vi "Feeder Move Arms.vi"(8 "error in (no error)":errorcluster, 11 "Action":enum16{"Drop", "Lift"}(ring)=enum."Lift") -> (0 "error out":errorcluster)   [LabVIEW 2014]
uses:
  Main/Robot Global Data.vi
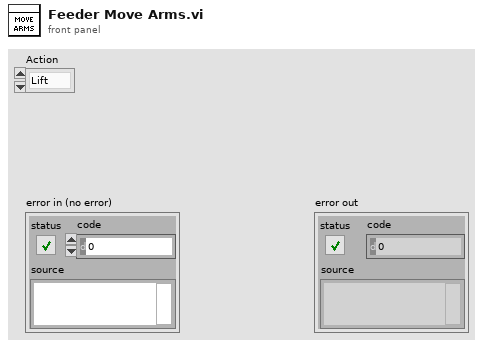
[diagram p1: front panel]
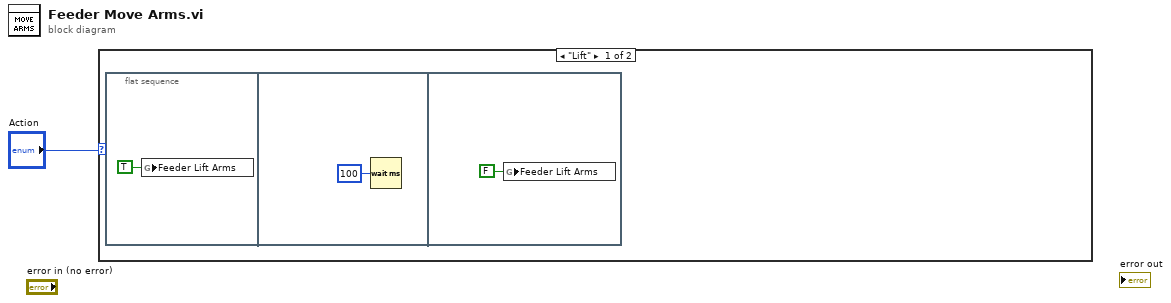
[diagram p0: block diagram]
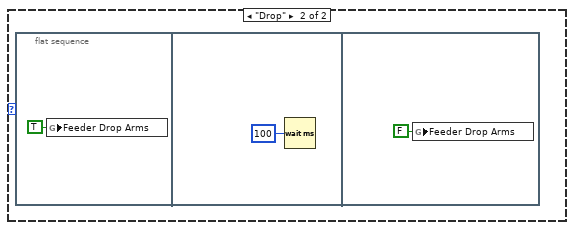
[diagram p2: hidden frame]
diagram:
  n1 = case shown="\"Lift\"" "Action" {
    frame "Lift" {
      n2 = flat-sequence {
        frame #0 {
          n3 = global write "Robot Global Data.vi" "Feeder Lift Arms"(TRUE ("Feeder Lift Arms")) -> ()
        }
        frame #1 {
          n4 = Wait (ms)(milliseconds to wait=u32 100) -> ()  [unwired: 1 out]
        }
        frame #2 {
          n5 = global write "Robot Global Data.vi" "Feeder Lift Arms"(FALSE ("Feeder Lift Arms")) -> ()
        }
      }
    }
    frame "Drop" {
      n6 = flat-sequence {
        frame #0 {
          n7 = global write "Robot Global Data.vi" "Feeder Drop Arms"(TRUE ("Feeder Lift Arms")) -> ()
        }
        frame #1 {
          n8 = Wait (ms)(milliseconds to wait=u32 100) -> ()  [unwired: 1 out]
        }
        frame #2 {
          n9 = global write "Robot Global Data.vi" "Feeder Drop Arms"(FALSE ("Feeder Lift Arms")) -> ()
        }
      }
    }
  }
